vi "display_custom_shortcut_menu.vi"(8 "error in (no error)":errorcluster, 9 "MenuRef":refnum<k9>, 10 "Ctl Refnum":refnum<vi>, 11 "TreeActorShortcutMenu in":refnum<class "TestEventFilter.lvclass">) -> (0 "error out":errorcluster, 2 "Discarded?":bool, 3 "TreeActorShortcutMenu out":refnum<class "TestEventFilter.lvclass">)   [LabVIEW 2015, in "TestViewables.lvlib" / "TestEventFilter.lvclass"]
uses:
  TestEventFilter.lvclass
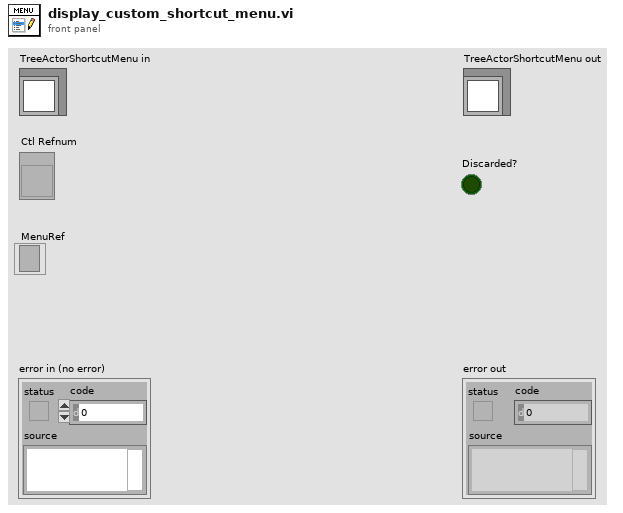
[diagram p1: front panel]
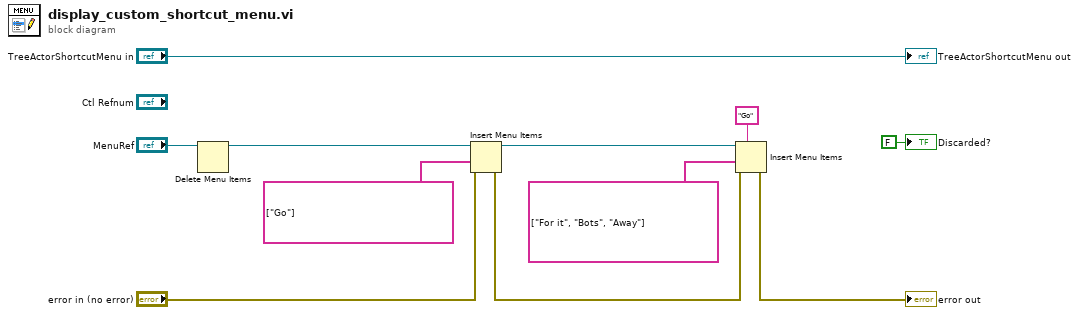
[diagram p0: block diagram]
diagram:
  n1 = Delete Menu Items(9:"MenuRef") -> (3:w2:refnum<k9>)  [unwired: 3 in, 1 out]
  n2 = Insert Menu Items(6:"error in (no error)", 7:string[] ["Go"] ("item tags"), 9:w2) -> (0:w4:errorcluster, 3:w7:refnum<k9>)  [unwired: 3 in, 1 out]
  n3 = Insert Menu Items(5:"Go" ("menu tag"), 6:w4, 7:string[] ["For it", "Bots", "Away"] ("item tags"), 9:w7) -> (0:→"error out":errorcluster)  [unwired: 2 in, 2 out]
  "TreeActorShortcutMenu out" <- "TreeActorShortcutMenu in"
  "Discarded?" <- FALSE ("Discarded?")
